vi "[CS] [Frame] Save to Davis File.vi"(8 "array":dbl[][](array[numeric]), 10 "Name":string, 11 "base path":path) -> ()   [LabVIEW 2014]
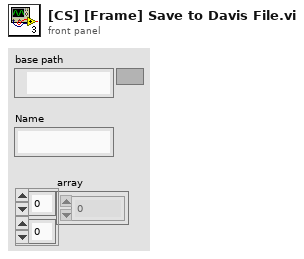
[diagram p1: front panel]
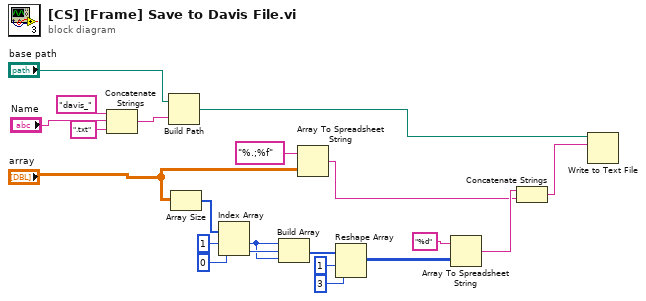
[diagram p0: block diagram]
diagram:
  n1 = Concatenate Strings("davis_" ("string"), "Name", ".txt" ("string")) -> (w6:string)
  n2 = Build Path(base path="base path", name or relative path=w6) -> (appended path=w9:path)
  n3 = Array Size(array="array") -> (size(s)=w16:i32[])
  n4 = Index Array(array=w16, index #1=1 ("index"), index #2=0 ("index")) -> (element #1=w12:i32, element #2=w13:i32)
  n5 = Build Array(w12, w13, w12) -> (w19:i32[])
  n6 = Array To Spreadsheet String(array="array", 3:"%.;%f" ("format string")) -> (spreadsheet string=w4:string)  [unwired: 1 in]
  n7 = Reshape Array(w19, 1 ("dimension size"), 3 ("dimension size")) -> (w10:i32[][])
  n8 = Array To Spreadsheet String(array=w10, 3:"%d" ("format string")) -> (spreadsheet string=w5:string)  [unwired: 1 in]
  n9 = Concatenate Strings(w5, w4) -> (w3:string)
  n10 = Write to Text File(file (use dialog)=w9, text=w3) -> ()  [unwired: 2 in, 3 out]
